vi "sourcemeter and signal analyzer3.vi"() -> ()   [LabVIEW 2018]
panel:
  out "output voltage":dbl[](array[numeric])
  in  "input voltage":dbl[](array[numeric])
  in  "Multiplier":dbl=1000000000000.0 format="%#_13e"
  in  "String 3":string="v_dn_21July.lvm"
  out "XY Graph":cluster{"Y":dbl[], "Y":dbl[]}[](graph)
  in  "String 2":string="v_dn_21July.lvm"
  in  "String1":string="N_2205_pressure_"
  in  "File Save Folder":path=path "D:/Soumen/OrbitalShaker/Pressure measurement/2205 particles/Run_21July/heating"
  in  "File save - yes/ no?":bool
  in  "No. of Measurements":i32=1000
  out "Save File Path":path
  out "Measure loop count":i32
  out "Voltage Loop count":i32
  out "Set Voltage":string
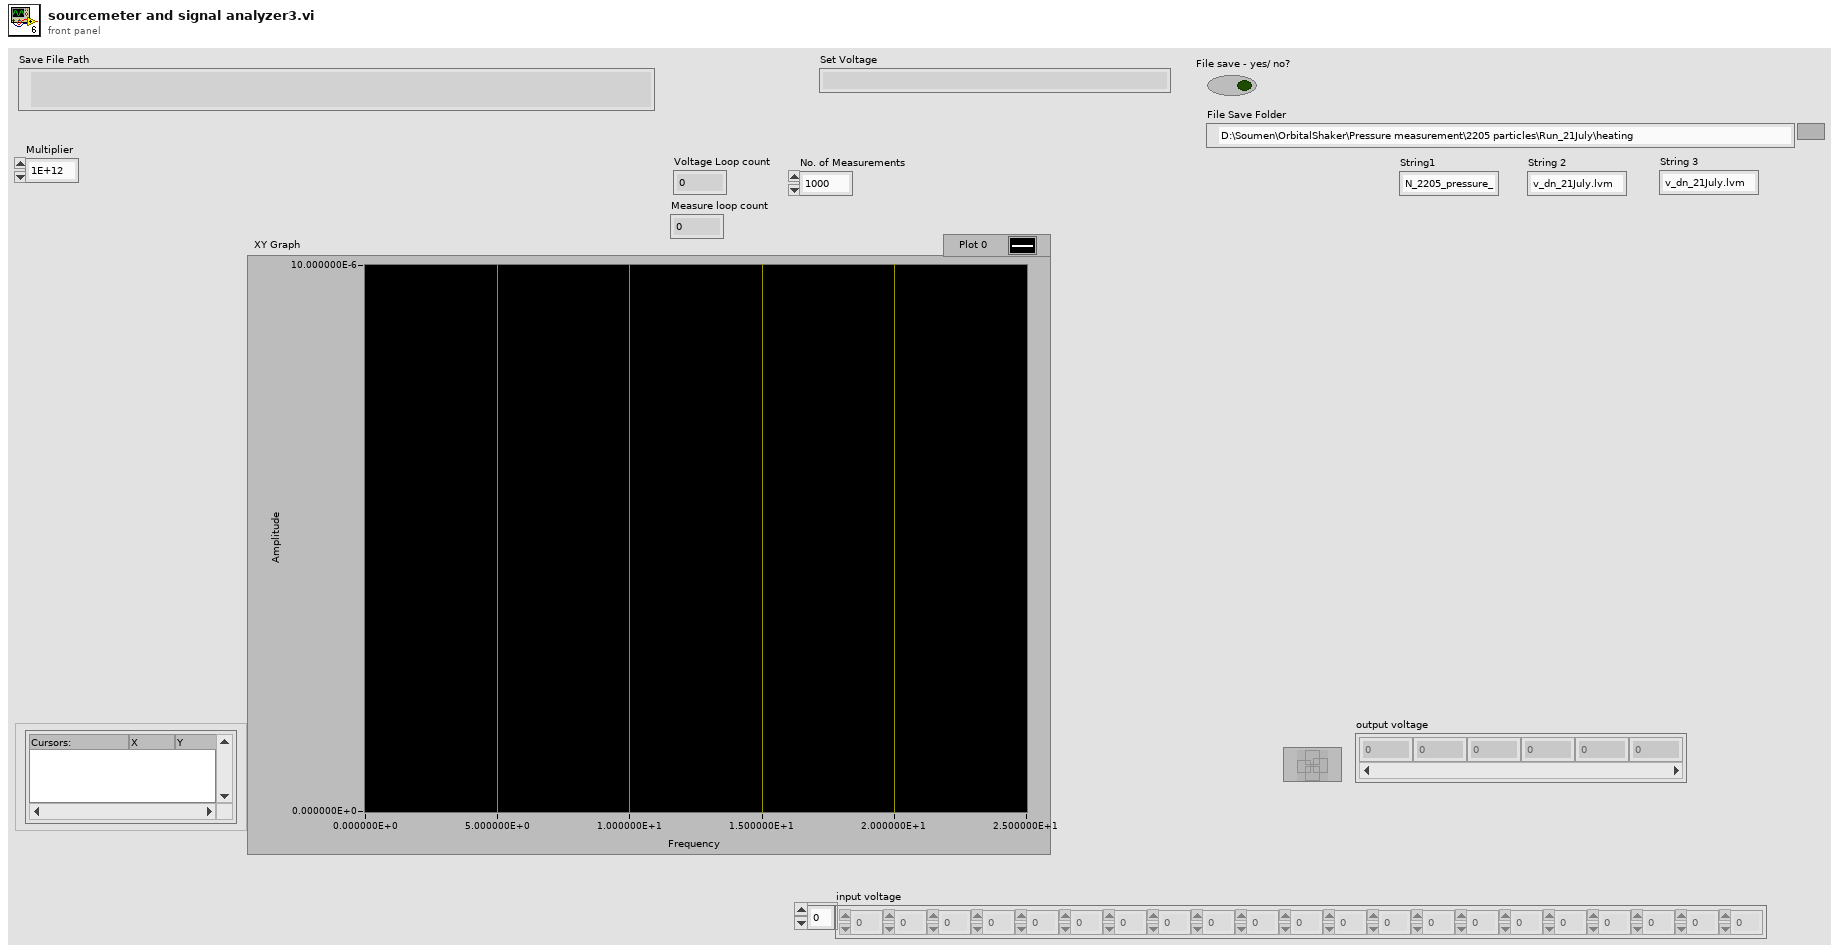
[diagram p1: front panel]
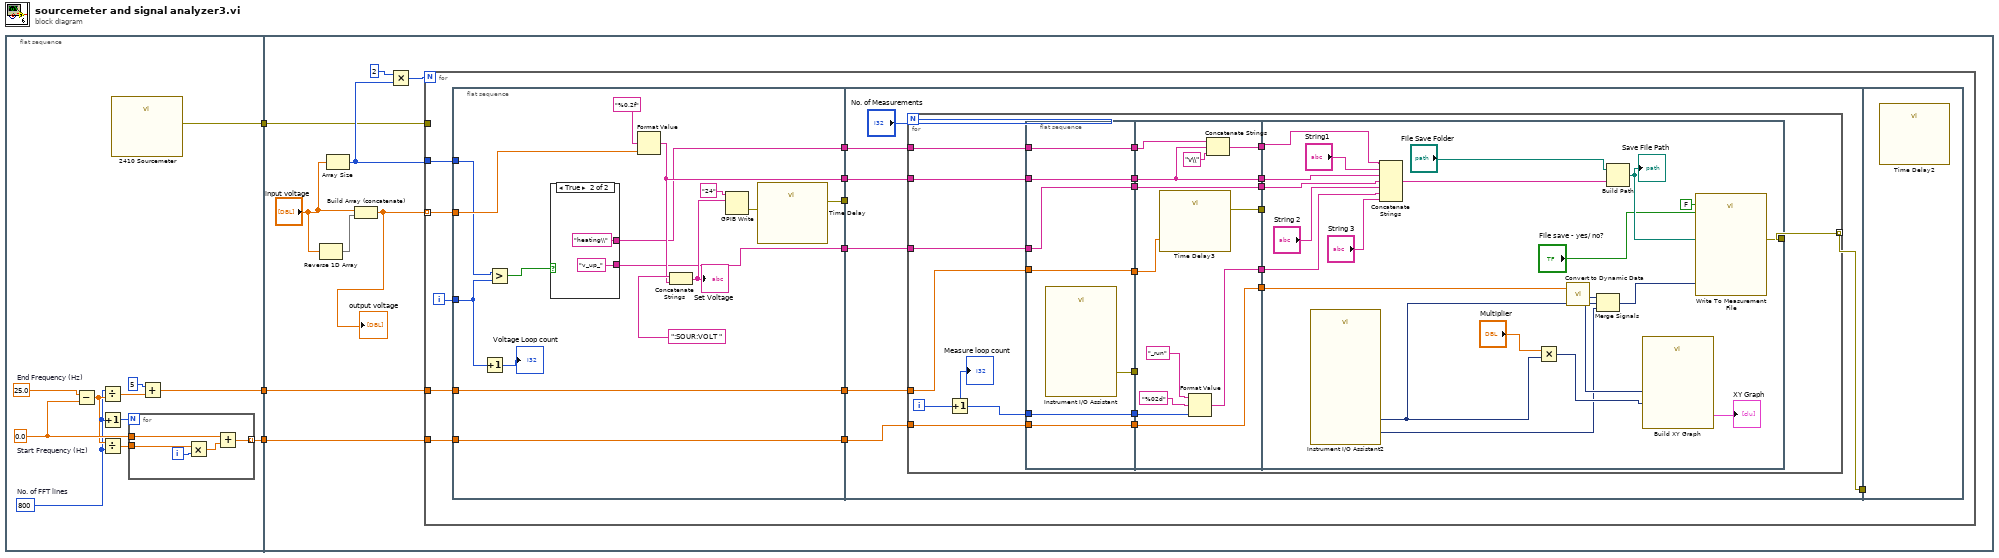
[diagram p0: block diagram]
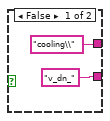
[diagram p2: hidden frame]
diagram:
  n1 = flat-sequence {
    tunnel: [w6] -> w3
    tunnel: [w5] -> w2
    tunnel: [w4] -> w1
    tunnel: w3 -> [w22]
    tunnel: w2 -> [w21]
    tunnel: w1 -> [w20]
    frame #0 {
      w14 = 25.0  # End Frequency (Hz)
      w8 = 800  # No. of FFT lines
      w13 = 0.0  # Start Frequency (Hz)
      n2 = Subtract(x=w14, y=w13) -> (x-y=w11:dbl)
      n3 = Divide(x=w8, y=w11) -> (x/y=w10:dbl)
      n4 = Increment(x=w8) -> (x+1=w7:i32)
      n5 = Divide(x=w11, y=w8) -> (x/y=w12:dbl)
      n6 = call "2410 Sourcemeter"() -> ("error out"=w4:errorcluster)  [unwired: 26 in, 1 out]
      n7 = for {
        N: w7 -> [_]
        tunnel: w13 -> [w19]
        tunnel: w12 -> [w17]
        tunnel: [w15] -> w5 mode=indexing
        i -> [w18]
        n8 = Multiply(x=w17, y=w18) -> (x*y=w16:dbl)
        n9 = Add(x=w19, y=w16) -> (x+y=w15:dbl)
      }
      n10 = Add(x=5, y=w10) -> (x+y=w6:dbl)
    }
    frame #1 {
      n11 = Reverse 1D Array(array="input voltage") -> (reversed array=w28:dbl[])
      n12 = Array Size(array="input voltage") -> (size(s)=w24:i32)
      n13 = Build Array (concatenate)("input voltage", w28) -> (w23:dbl[])
      "output voltage" <- w23
      n14 = Multiply(x=2, y=w24) -> (x*y=w25:i32)
      n15 = for {
        N: w25 -> [_]
        tunnel: w22 -> [w36]
        tunnel: w21 -> [w34]
        tunnel: w24 -> [w30]
        tunnel: w23 -> [w29] mode=indexing
        tunnel: w20 -> [_]
        i -> [w40]
        n16 = flat-sequence {
          tunnel: w40 -> [w42]
          tunnel: [w51] -> w38
          tunnel: [w50] -> w37
          tunnel: w36 -> [w50]
          tunnel: [w49] -> w35
          tunnel: w34 -> [w49]
          tunnel: [w48] -> w33
          tunnel: [w47] -> w32
          tunnel: [w45] -> w31
          tunnel: w30 -> [w43]
          tunnel: w29 -> [w44]
          tunnel: [w66] -> w39
          tunnel: w38 -> [w65]
          tunnel: w37 -> [w64]
          tunnel: w35 -> [w63]
          tunnel: w33 -> [w62]
          tunnel: w32 -> [w61]
          tunnel: w31 -> [_]
          tunnel: w39 -> [_]
          frame #0 {
            n17 = Increment(x=w42) -> (x+1=→"Voltage Loop count":i32)
            n18 = Greater?(x=w43, y=w42) -> (0:w41:bool)
            n19 = case shown="True" w41 {
              tunnel: ["cooling\\" "heating\\"] -> w48
              tunnel: ["v_dn_" "v_up_"] -> w47
              frame False {
              }
              frame True {
              }
            }
            n20 = Format Value(format string="%0.2f", value (0)=w44) -> (output string=w51:string)  [unwired: 1 in]
            n21 = Concatenate Strings(":SOUR:VOLT ", w51) -> (w52:string)
            "Set Voltage" <- w52
            n22 = GPIB Write(0:"24" ("address string"), 1:w52) -> (6:w53:errorcluster)  [unwired: 3 in, 1 out]
            n23 = call "Time Delay"("error in (no error)"=w53) -> ("error out"=w45:errorcluster)  [unwired: 10 in]
          }
          frame #1 {
            n24 = for {
              N: "No. of Measurements" -> [_]
              tunnel: [w88] -> w66 mode=indexing
              tunnel: w65 -> [w80]
              tunnel: w64 -> [w86]
              tunnel: w63 -> [w85]
              tunnel: w62 -> [w74]
              tunnel: w61 -> [w72]
              i -> [w69]
              n25 = Increment(x=w69) -> (x+1=w68:i32)
              "Measure loop count" <- w68
              n26 = flat-sequence {
                tunnel: [w95] -> w87
                tunnel: w86 -> [w95]
                tunnel: w85 -> [w94]
                tunnel: [w94] -> w83
                tunnel: [w93] -> w81
                tunnel: w80 -> [w93]
                tunnel: [w92] -> w79
                tunnel: w68 -> [w92]
                tunnel: [w91] -> w76
                tunnel: [w90] -> w75
                tunnel: w74 -> [w90]
                tunnel: [w89] -> w73
                tunnel: w72 -> [w89]
                tunnel: w87 -> [w107]
                tunnel: [w106] -> w84
                tunnel: w83 -> [w106]
                tunnel: [w100] -> w82
                tunnel: w81 -> [w100]
                tunnel: w79 -> [w105]
                tunnel: [w104] -> w78
                tunnel: [w101] -> w77
                tunnel: w76 -> [_]
                tunnel: w75 -> [w98]
                tunnel: w73 -> [w97]
                tunnel: [w97] -> w71
                tunnel: [w96] -> w70
                tunnel: [w128] -> w88
                tunnel: w84 -> [w116]
                tunnel: w82 -> [w109]
                tunnel: w78 -> [w114]
                tunnel: w77 -> [w112]
                tunnel: w71 -> [w110]
                tunnel: w70 -> [_]
                frame #0 {
                  n27 = call "Instrument I/O Assistant"() -> ("error out"=w91:errorcluster)  [unwired: 26 in, 1 out]
                }
                frame #1 {
                  n28 = call "Time Delay3"("Delay Time (s)"=w107) -> ("error out"=w96:errorcluster)  [unwired: 10 in]
                  n29 = Format Value(string ("")="_run" ("format string"), format string="%02d" ("format string 2"), value (0)=w105) -> (output string=w104:string)
                  n30 = Concatenate Strings(w98, w100, "v\\" ("string")) -> (w101:string)
                }
                frame #2 {
                  n31 = call "Instrument I/O Assistant2"() -> ("token2"=w108:dynamicdata, "token"=w119:dynamicdata)  [unwired: 24 in, 2 out]
                  n32 = Concatenate Strings(w112, "String1", w109, w110, "String 2", w114, "String 3") -> (w125:string)
                  n33 = Multiply(x="Multiplier", y=w119) -> (x*y=w117:dynamicdata)
                  n34 = call "Convert to Dynamic Data"("Array"=w116) -> ("Dynamic Data Type"=w113:dynamicdata)  [unwired: 3 in]
                  n35 = Merge Signals(w113, w119, w108) -> (w120:dynamicdata)
                  n36 = Build Path(base path="File Save Folder", name or relative path=w125) -> (appended path=w124:path)
                  "Save File Path" <- w124
                  n37 = call "Build XY Graph"("Y Input"=w117, "X Input"=w113) -> ("XY Graph"=→"XY Graph":cluster{"X":dbl[], "Y":dbl[]}[])  [unwired: 8 in, 1 out]
                  n38 = call "Write To Measurement File"("Signals"=w120, "Reset"=FALSE, "Enable"="File save - yes/ no?", "Filename"=w124) -> ("error out"=w128:errorcluster)  [unwired: 13 in, 2 out]
                }
              }
            }
          }
          frame #2 {
            n39 = call "Time Delay2"() -> ()  [unwired: 11 in, 1 out]
          }
        }
      }
    }
  }
